vi "10_2.vi"() -> ()   [LabVIEW 2025, in "2022.lvlib"]
uses:
  2022.lvlib
panel:
  out "appended array":string[](array[string])
  out "Array 3":string[][](array[string])
  out "Array 2":i32[](array[numeric])
  out "sum":i32
  out "Array":i32[](array[numeric])
  out "output 2":i32
  out "Numeric":i32
  out "delimiter":string
  # "PZGPKPEB"
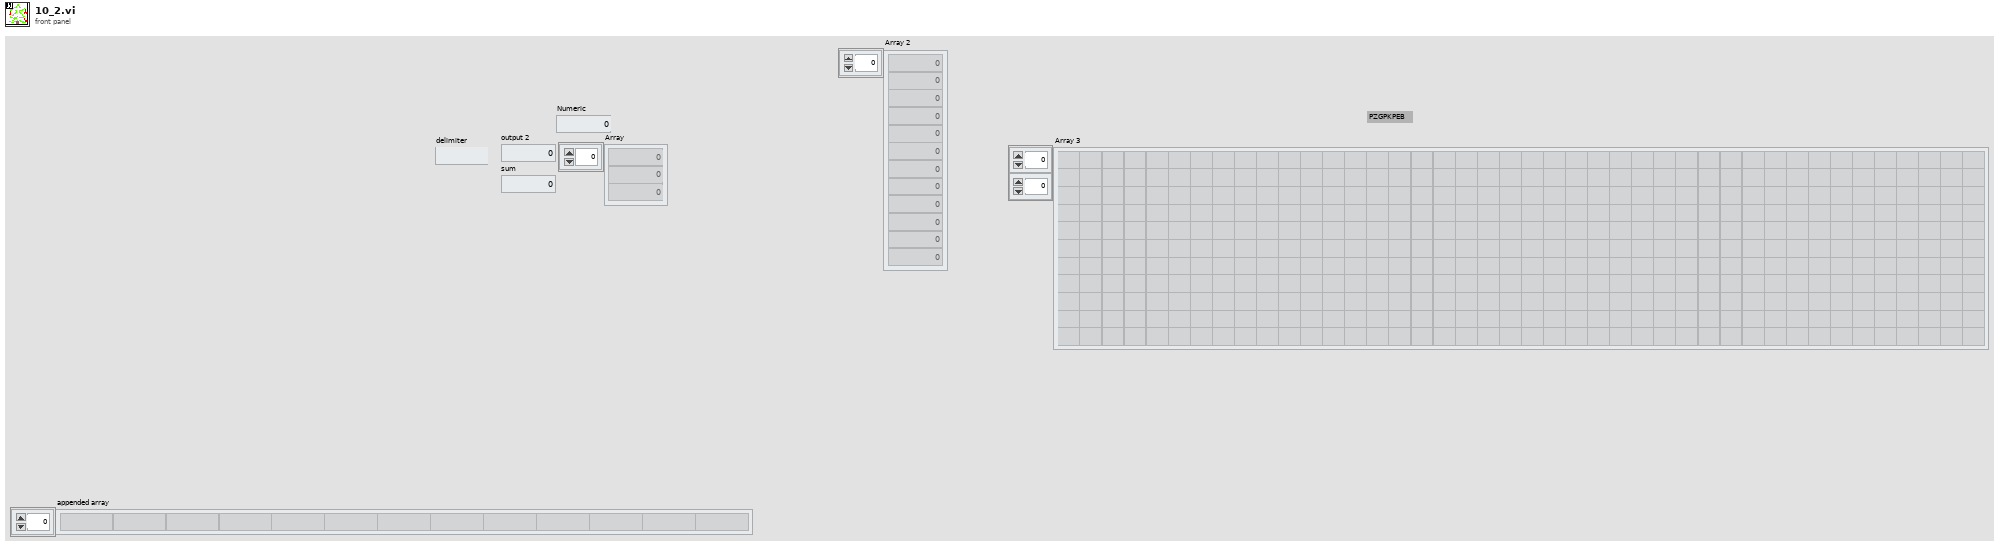
[diagram p1: front panel]
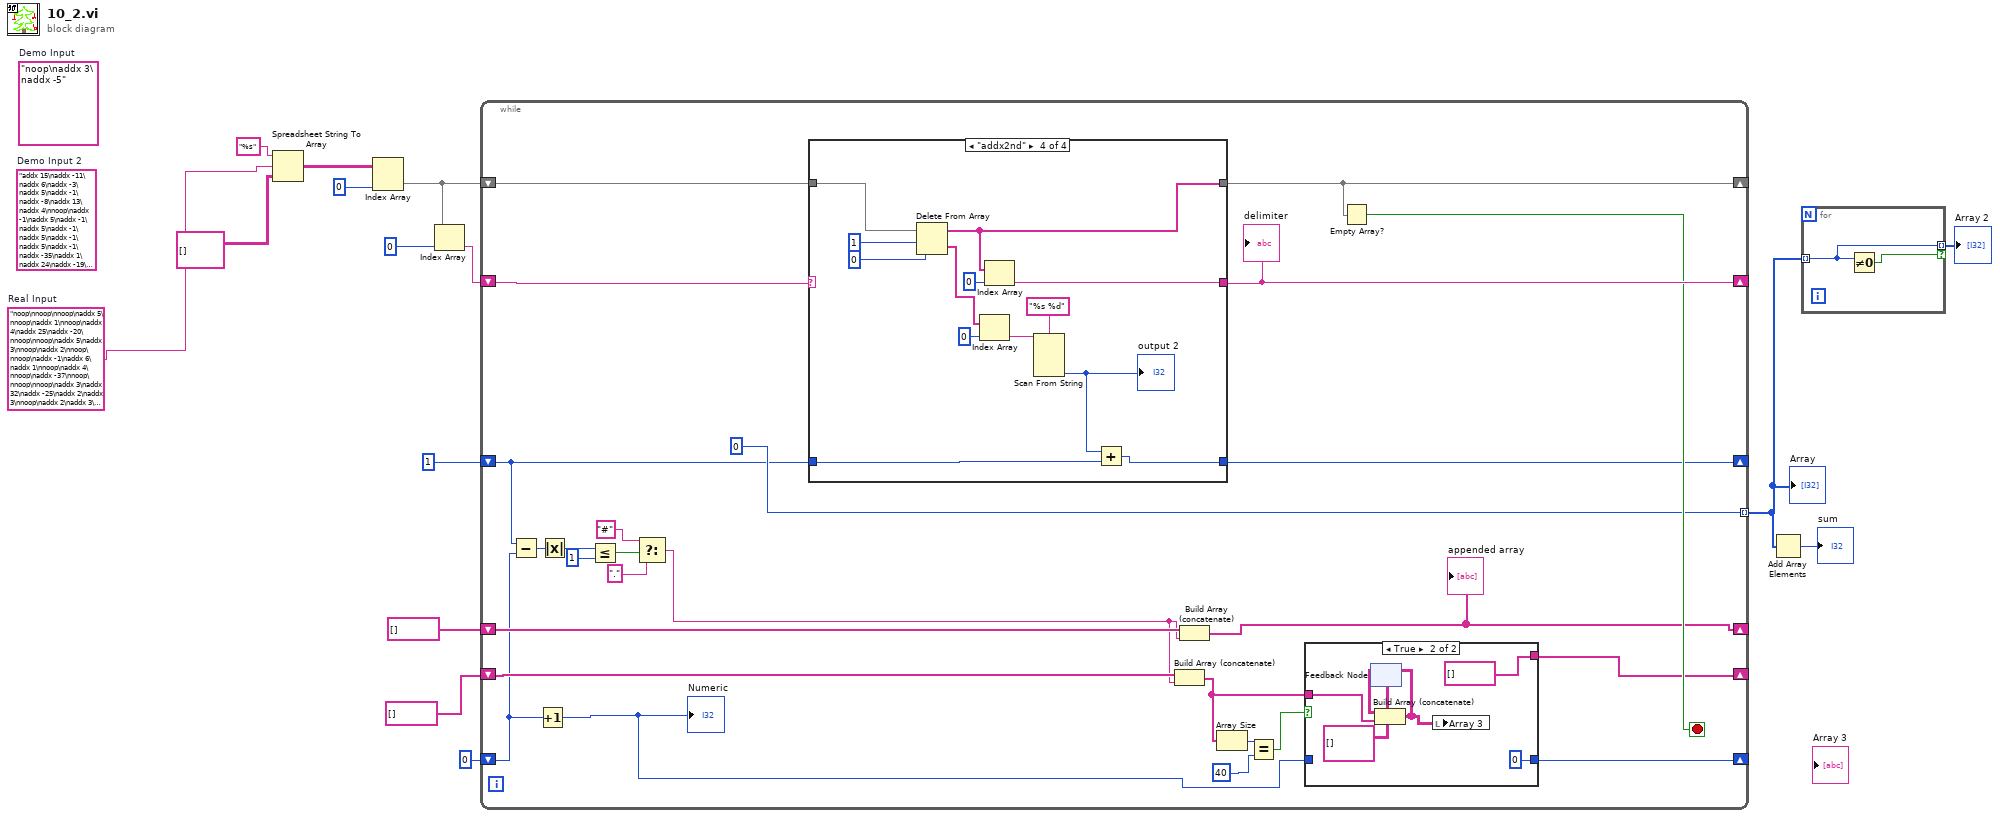
[diagram p0: block diagram]
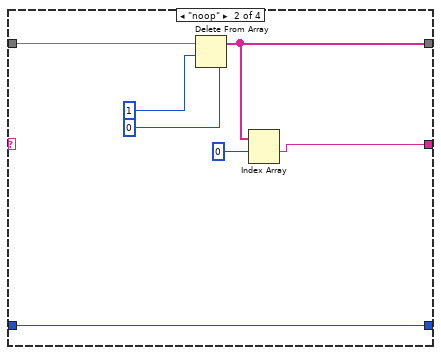
[diagram p4: hidden frame]
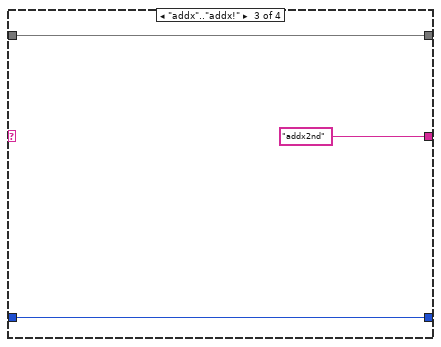
[diagram p5: hidden frame]
diagram:
  (unwired) "addx 15\naddx -11\naddx 6\naddx -3\naddx 5\naddx -1\naddx -8\naddx 13\naddx 4\nnoop\naddx -1\naddx 5\naddx -1\naddx 5\naddx -1\naddx 5\naddx -1\naddx 5\naddx -1\naddx -35\naddx 1\naddx 24\naddx -19\naddx 1\naddx 16\naddx -11\nnoop\nnoop\naddx 21\naddx -15\nnoop\nnoop\naddx -3\naddx 9\naddx 1\naddx -3\naddx 8\naddx 1\naddx 5\nnoop\nnoop\nnoop\nnoop\nnoop\naddx -36\nnoop\naddx 1\naddx 7\nnoop\nnoop\nnoop\naddx 2\naddx 6\nnoop\nnoop\nnoop\nnoop\nnoop\naddx 1\nnoop\nnoop\naddx 7\naddx 1\nnoop\naddx -13\naddx 13\naddx 7\nnoop\naddx 1\naddx -33\nnoop\nnoop\nnoop\naddx 2\nnoop\nnoop\nnoop\naddx 8\nnoop\naddx -1\naddx 2\naddx 1\nnoop\naddx 17\naddx -9\naddx 1\naddx 1\naddx -3\naddx 11\nnoop\nnoop\naddx 1\nnoop\naddx 1\nnoop\nnoop\naddx -13\naddx -19\naddx 1\naddx 3\naddx 26\naddx -30\naddx 12\naddx -1\naddx 3\naddx 1\nnoop\nnoop\nnoop\naddx -9\naddx 18\naddx 1\naddx 2\nnoop\nnoop\naddx 9\nnoop\nnoop\nnoop\naddx -1\naddx 2\naddx -37\naddx 1\naddx 3\nnoop\naddx 15\naddx -21\naddx 22\naddx -6\naddx 1\nnoop\naddx 2\naddx 1\nnoop\naddx -10\nnoop\nnoop\naddx 20\naddx 1\naddx 2\naddx 2\naddx -6\naddx -11\nnoop\nnoop\nnoop"  # Demo Input 2
  w1 = "noop\nnoop\nnoop\naddx 5\nnoop\naddx 1\nnoop\naddx 4\naddx 25\naddx -20\nnoop\nnoop\naddx 5\naddx 3\nnoop\naddx 2\nnoop\nnoop\naddx -1\naddx 6\naddx 1\nnoop\naddx 4\nnoop\naddx -37\nnoop\nnoop\nnoop\naddx 3\naddx 32\naddx -25\naddx 2\naddx 3\nnoop\naddx 2\naddx 3\nnoop\naddx 2\naddx 2\naddx -24\naddx 25\naddx 5\naddx 2\naddx 8\naddx -23\naddx 18\naddx 5\naddx -39\naddx 11\naddx -9\naddx 6\naddx -2\naddx 5\naddx 4\naddx -4\naddx 3\naddx 5\naddx 2\nnoop\naddx -1\naddx 6\naddx -21\naddx 22\naddx 3\naddx 1\naddx 5\nnoop\nnoop\naddx -35\nnoop\nnoop\nnoop\nnoop\naddx 37\naddx -33\nnoop\naddx 6\naddx 2\naddx -1\naddx 3\naddx 1\naddx 5\naddx 2\naddx -19\naddx 21\naddx 1\naddx 5\naddx -31\naddx 36\nnoop\naddx 3\naddx -2\naddx -38\nnoop\nnoop\naddx 7\naddx 14\naddx -4\naddx -7\naddx 5\naddx 2\naddx 12\naddx -15\naddx 6\naddx 2\naddx 5\naddx -27\naddx 25\naddx 5\nnoop\naddx 7\naddx -2\naddx 5\naddx -40\nnoop\naddx 7\nnoop\naddx -1\naddx 2\naddx 5\naddx -1\naddx 1\naddx 2\naddx 7\nnoop\naddx -2\nnoop\naddx 3\naddx 2\naddx 7\nnoop\nnoop\naddx 1\nnoop\nnoop\naddx 3\naddx 1\nnoop\nnoop\nnoop"  # Real Input
  (unwired) "noop\naddx 3\naddx -5"  # Demo Input
  n1 = Spreadsheet String To Array(format string="%s", spreadsheet string=w1, array type (2D Dbl)=string[][] []) -> (array=w13:string[][])  [unwired: 1 in]
  n2 = Index Array(array=w13, index (col)=0 ("index (row)")) -> (element=w12:string[])  [unwired: 1 in]
  n3 = Index Array(array=w12, index=0) -> (element=w11:string)
  n4 = while {
    shift-right: [w38] -> _
    shift-left: w12 -> [w41]
    shift-right: [w39] -> _
    shift-left: w11 -> [w40]
    shift-right: [w27] -> _
    shift-left: 1 ("Numeric") -> [w28]
    tunnel: [0] -> w6 mode=indexing
    shift-right: [w25] -> _
    shift-left: string[] [] -> [w32]
    shift-right: [w26] -> _
    shift-left: string[] [] -> [w21]
    shift-right: [w18] -> _
    shift-left: 0 -> [w16]
    stop <- w37 stop-if-true
    n5 = Subtract(x=w28, y=w16) -> (x-y=w34:i32)
    n6 = Increment(x=w16) -> (x+1=w17:i32)
    "Numeric" <- w17
    n7 = Absolute Value(x=w34) -> (abs(x)=w35:i32)
    n8 = Less Or Equal?(x=w35, y=1) -> (x <= y?=w31:bool)
    n9 = Select(t="#" ("delimiter"), s=w31, f=".") -> (s? t:f=w20:string)
    n10 = case shown="\"addx2nd\"" w40 {
      selector: w40 -> [w51 _ _ _]
      tunnel: w41 -> [w52 w59 w62 w72]
      tunnel: [w52 w55 w62 w71] -> w38
      tunnel: [w51 w54 "addx2nd" ("delimiter") w69] -> w39
      tunnel: w28 -> [w50 w53 w60 w67]
      tunnel: [w50 w53 w60 w66] -> w27
      frame "False", Default {
      }
      frame "noop" {
        n11 = Delete From Array(array=w59, length=1, index=0) -> (array with subset deleted=w55:string[])  [unwired: 1 out]
        n12 = Index Array(array=w55, index #1=0 ("index")) -> (element #1=w54:string)  [unwired: 1 in, 1 out]
      }
      frame "addx".."addx!" {
      }
      frame "addx2nd" {
        n13 = Delete From Array(array=w72, length=1, index=0) -> (deleted portion=w64:string[], array with subset deleted=w71:string[])
        n14 = Index Array(array=w64, index=0) -> (element=w63:string)
        n15 = Index Array(array=w71, index=0) -> (element=w69:string)
        n16 = Scan From String(format string="%s %d", input string=w63) -> (output 2=w68:i32)  [unwired: 5 in, 3 out]
        "output 2" <- w68
        n17 = Add(x=w68, y=w67) -> (x+y=w66:i32)
      }
    }
    "delimiter" <- w39
    n18 = Build Array (concatenate)(w21, w20) -> (w19:string[])
    n19 = Build Array (concatenate)(w32, w20) -> (w25:string[])
    "appended array" <- w25
    n20 = Array Size(array=w19) -> (size(s)=w24:i32)
    n21 = Equal?(x=w24, y=40) -> (x = y?=w22:bool)
    n22 = case shown="True" w22 {
      tunnel: w19 -> [w43 w47]
      tunnel: [w43 string[] []] -> w26
      tunnel: [w42 0] -> w18
      tunnel: w17 -> [w42 _]
      frame False {
      }
      frame True {
        n23 = feedback #1(string[][] []) -> (w48:string[][])
        n24 = Build Array (concatenate)(w48, w47) -> (w45:string[][])
        n25 = feedback-in #1(w45) -> ()
        n26 = local write "Array 3"(w45) -> ()
      }
    }
    n27 = Empty Array?(array=w38) -> (empty?=w37:bool)
  }
  "Array" <- w6
  n28 = Add Array Elements(numeric array=w6) -> (sum=→"sum":i32)
  n29 = for {
    tunnel: w6 -> [w77] mode=indexing
    tunnel: [w77] -> w5 mode=indexing if=w76
    n30 = Not Equal To 0?(x=w77) -> (x != 0?=w76:bool)
  }
  "Array 2" <- w5
